vi "KtoC.vi"() -> ()   [LabVIEW 2022 SP3]
uses:
  Kcotoo.vi
panel:
  out "x+y":dbl
  in  "C":dbl
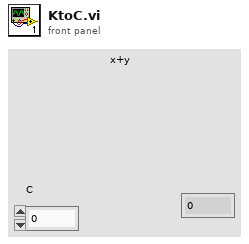
[diagram p1: front panel]
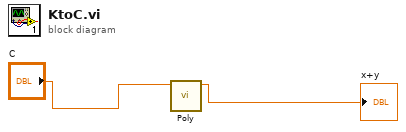
[diagram p0: block diagram]
diagram:
  n1 = call-poly "Poly.vi"("C"="C") -> ("Numeric"=→"x+y":dbl)  [unwired: 10 in]
